vi "Begin.vi"(8 "error in":errorcluster) -> (0 "error out":errorcluster)   [LabVIEW 2017]
doc: "Called before other user functions, this VI is expected to open initial I/O refnums, load in file data, and do all program initialization. Notice that the <B>error out</B> terminal is simply used for data flow. Wiring it to other structures or subVIs ensures that this VI runs first."
uses:
  <vilib>/Rock Robotics/WPI/DriverStation/WPI_DriverStationRobotMode2.ctl
  TypeDef/CLUSTER_Claw_Setup.ctl
  TypeDef/CLUSTER_PWM Motor Setup.ctl
  <vilib>/Rock Robotics/SystemInterfaces/DIO/FPGA_DIOPWMChannel.ctl
  Robot Global Data.vi
  _SHARE ALL/Global Share All/Global_STOP.vi
  Globals/Global_Device_IDs.vi
  System Drivers/Phoenix-LabVIEW/Motor Controller/Controls/CTRE_Phoenix_MotorControl_FeedbackDevice.ctl
  TypeDef/CLUSTER_PID.ctl
  TypeDef/CLUSTER_Talon_Setup.ctl
  TypeDef/CLUSTER_Arm_Device_IDs.ctl
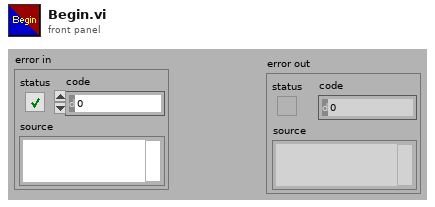
[diagram p1: front panel]
types:
  T1 = typedef "FPGA_DIOPWMChannel.ctl" = enum8{"PWM 0", "PWM 1", "PWM 2", "PWM 3", "PWM 4", "PWM 5", "PWM 6", "PWM 7", "PWM 8", "PWM 9", "PWM MXP 0", "PWM MXP 1", "PWM MXP 2", "PWM MXP 3", "PWM MXP 4", "PWM MXP 5", "PWM MXP 6", "PWM MXP 7", "PWM MXP 8", "PWM MXP 9", "Invalid"}
  T2 = typedef "CLUSTER_Claw_Setup.ctl" = cluster{"Left Motor Setup":T3, "Right Motor Setup":T3}
  T3 = typedef "CLUSTER_PWM Motor Setup.ctl" = cluster{"Motor PWM":T1, "Invert Motor":bool}
  T4 = typedef "WPI_DriverStationRobotMode2.ctl" = enum16{"Autonomous Disabled", "Autonomous Enabled", "Teleop Disabled", "Teleop Enabled", "Disconnected", "Finish", "Test Disabled", "Test Enabled", "Emergency Stopped"}
  T5 = typedef "CLUSTER_Talon_Setup.ctl" = cluster{"Talon SRX ID":u8, "PhaseSensor":bool, "Invert Motor?":bool, "Phoenix Feedback Select":T6, "pidLoopldx":i32, "PID":T7}
  T6 = typedef "CTRE_Phoenix_MotorControl_FeedbackDevice.ctl" = i8
  T7 = typedef "CLUSTER_PID.ctl" = cluster{"P":dbl, "I":dbl, "D":dbl, "F":dbl, "I Zone":dbl}
  T8 = typedef "CLUSTER_Arm_Device_IDs.ctl" = cluster{"Elbow Setup":T5, "Telescope Setup":T5, "Wrist Setup":T5}
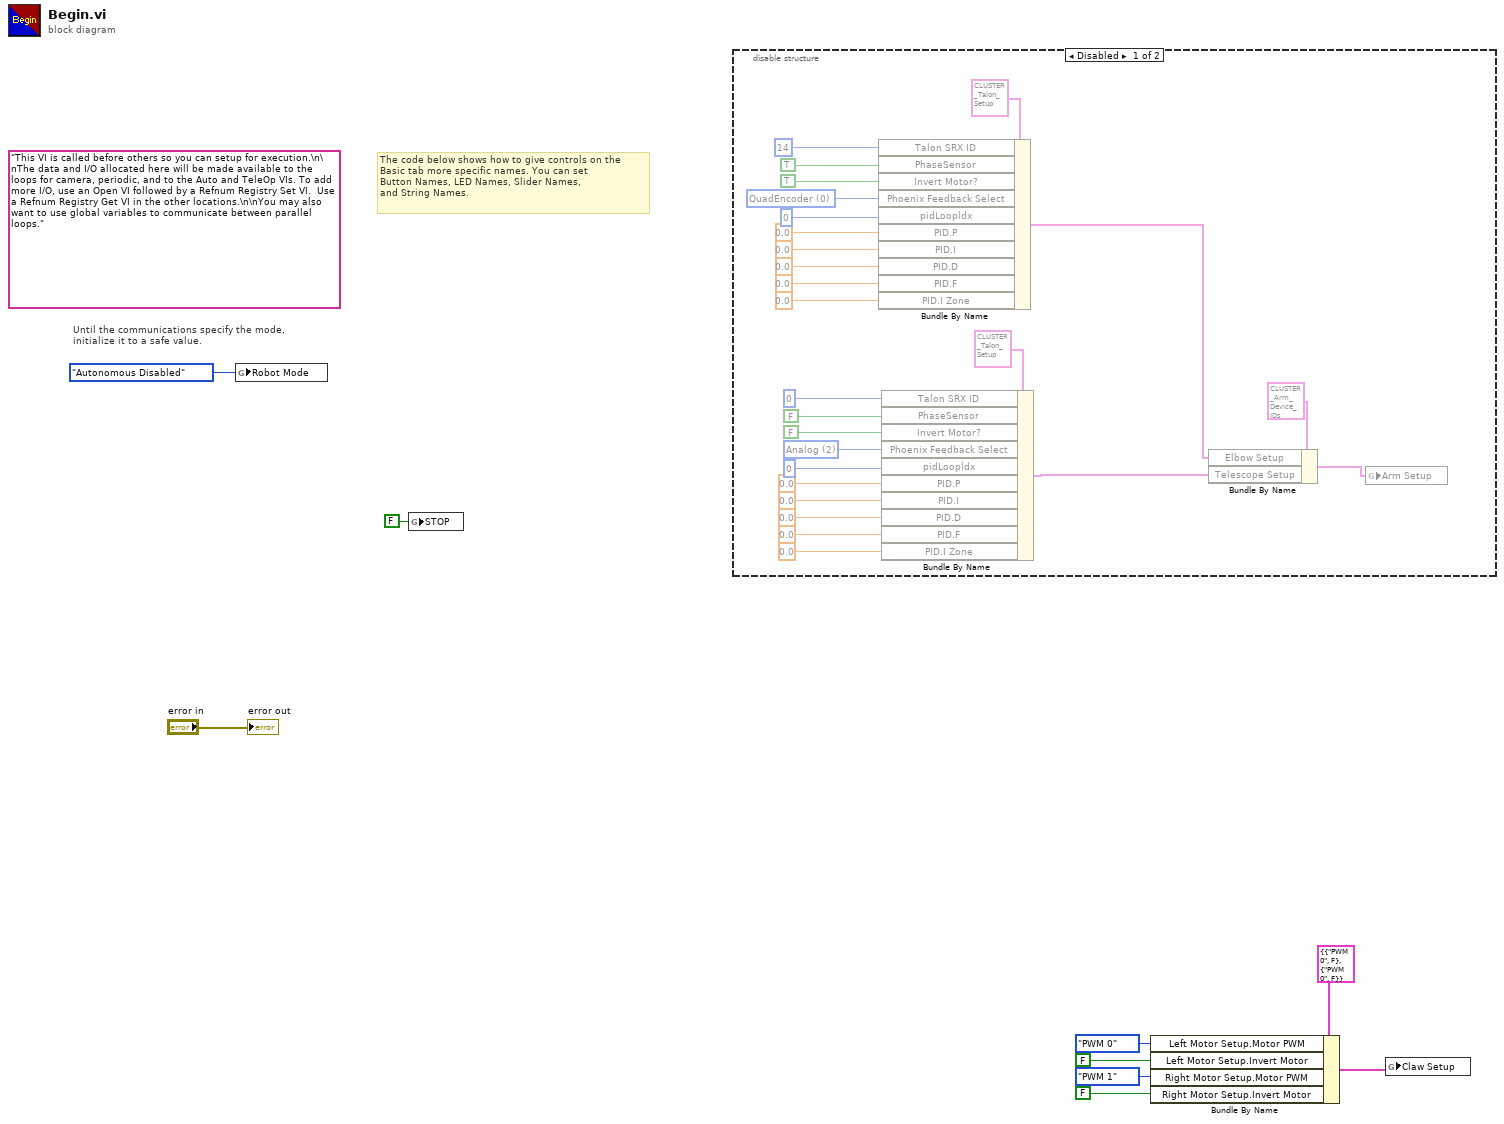
[diagram p0: block diagram]
diagram:
  (unwired) "This VI is called before others so you can setup for execution.\n\nThe data and I/O allocated here will be made available to the loops for camera, periodic, and to the Auto and TeleOp VIs. To add more I/O, use an Open VI followed by a Refnum Registry Set VI.  Use a Refnum Registry Get VI in the other locations.\n\nYou may also want to use global variables to communicate between parallel loops."
  # "The code below shows how to give controls on the\nBasic tab more specific names. You can set\nButton Names, LED Names, Slider Names,\nand String Names."
  # "Until the communications specify the mode,\ninitialize it to a safe value."
  n1 = global write "Robot Global Data.vi" "Robot Mode"(WPI_DriverStationRobotMode2."Autonomous Disabled" ("Robot Mode")) -> ()
  n2 = global write "Global_STOP.vi" "STOP"(FALSE ("STOP")) -> ()
  n3 = disable-structure shown="Disabled" {
    frame Disabled {
      w17 = T6 2 items=["None"=-1, "QuadEncoder"=0, "Analog"=2, "Tachometer"=4, "Pulse Width Encoded Position"=8, "Sensor Sum (S0 + S1)"=9, "Sensor Difference (D0 - D1)"=10, "Remote Source 0"=11, "Remote Source 1"=12, "Software Emulated"=15] ("Phoenix Feedback Select")
      w30 = T6 0 items=["None"=-1, "QuadEncoder"=0, "Analog"=2, "Tachometer"=4, "Pulse Width Encoded Position"=8, "Sensor Sum (S0 + S1)"=9, "Sensor Difference (D0 - D1)"=10, "Remote Source 0"=11, "Remote Source 1"=12, "Software Emulated"=15] ("Phoenix Feedback Select")
      n4 = Bundle By Name(cluster=T5 {"Talon SRX ID"=0, "PhaseSensor"=FALSE, "Invert Motor?"=FALSE, "Phoenix Feedback Select"=-1, "pidLoopldx"=0, "PID"={"P"=0.0, "I"=0.0, "D"=0.0, "F"=0.0, "I Zone"=0.0}} ("Elbow Setup"), "Talon SRX ID"=u8 14, "PhaseSensor"=TRUE, "Invert Motor?"=TRUE, "Phoenix Feedback Select"=w30, "pidLoopldx"=0, "PID.P"=0.0, "PID.I"=0.0, "PID.D"=0.0, "PID.F"=0.0, "PID.I Zone"=0.0) -> (w11:T5)
      n5 = Bundle By Name(cluster=T5 {"Talon SRX ID"=0, "PhaseSensor"=FALSE, "Invert Motor?"=FALSE, "Phoenix Feedback Select"=-1, "pidLoopldx"=0, "PID"={"P"=0.0, "I"=0.0, "D"=0.0, "F"=0.0, "I Zone"=0.0}} ("Elbow Setup"), "Talon SRX ID"=u8 0, "PhaseSensor"=FALSE, "Invert Motor?"=FALSE, "Phoenix Feedback Select"=w17, "pidLoopldx"=0, "PID.P"=0.0, "PID.I"=0.0, "PID.D"=0.0, "PID.F"=0.0, "PID.I Zone"=0.0) -> (w12:T5)
      n6 = Bundle By Name(cluster=T8 {"Elbow Setup"={"Talon SRX ID"=0, "PhaseSensor"=FALSE, "Invert Motor?"=FALSE, "Phoenix Feedback Select"=2, "pidLoopldx"=0, "PID"={"P"=0.0, "I"=0.0, "D"=0.0, "F"=0.0, "I Zone"=0.0}}, "Telescope Setup"={"Talon SRX ID"=0, "PhaseSensor"=FALSE, "Invert Motor?"=FALSE, "Phoenix Feedback Select"=-1, "pidLoopldx"=0, "PID"={"P"=0.0, "I"=0.0, "D"=0.0, "F"=0.0, "I Zone"=0.0}}, "Wrist Setup"={"Talon SRX ID"=0, "PhaseSensor"=FALSE, "Invert Motor?"=FALSE, "Phoenix Feedback Select"=-1, "pidLoopldx"=0, "PID"={"P"=0.0, "I"=0.0, "D"=0.0, "F"=0.0, "I Zone"=0.0}}} ("Arm Setup"), "Elbow Setup"=w11, "Telescope Setup"=w12) -> (w10:T8)
      n7 = global write "Global_Device_IDs.vi" "Arm Setup"(w10) -> ()
    }
    frame Enabled {
    }
  }
  n8 = Bundle By Name(cluster=T2 {"Left Motor Setup"={"Motor PWM"=enum."PWM 0", "Invert Motor"=FALSE}, "Right Motor Setup"={"Motor PWM"=enum."PWM 0", "Invert Motor"=FALSE}} ("Claw Setup"), "Left Motor Setup.Motor PWM"=FPGA_DIOPWMChannel."PWM 0", "Left Motor Setup.Invert Motor"=FALSE, "Right Motor Setup.Motor PWM"=FPGA_DIOPWMChannel."PWM 1", "Right Motor Setup.Invert Motor"=FALSE) -> (w5:T2)
  n9 = global write "Global_Device_IDs.vi" "Claw Setup"(w5) -> ()
  "error out" <- "error in"
